vi "LED-Change text.vi"(6 "Container State":T1, 7 "LED Display":refnum<vi>, 8 "error in (no error)":errorcluster, 9 "Should Change?":bool, 10 "Data In":T2, 11 "vi reference in":refnum<vi>) -> (0 "error out":errorcluster, 2 "Data Out":T2, 3 "vi reference out":refnum<vi>)   [LabVIEW 2012, in "LED Display.xctl"]
doc: "This VI changes the text to be displayed in the LED XControl"
uses:
  LED Display.xctl
  LED-Data.ctl
  <vilib>/_xctls/Container State.ctl
  <vilib>/_xctls/XControlSupport.lvlib
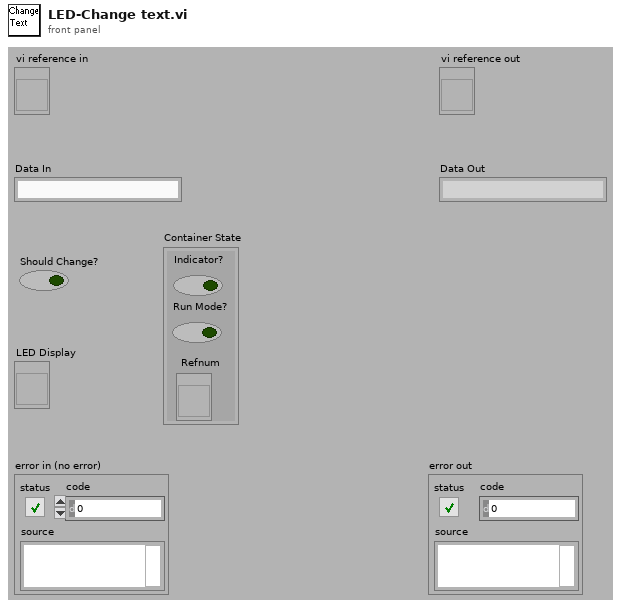
[diagram p1: front panel]
types:
  T1 = typedef "XControlSupport.lvlib/Container State.ctl" = cluster{"Indicator?":bool, "Run Mode?":bool, " Refnum":refnum<vi>}
  T2 = typedef "LED Display.xctl/LED-Data.ctl" = string
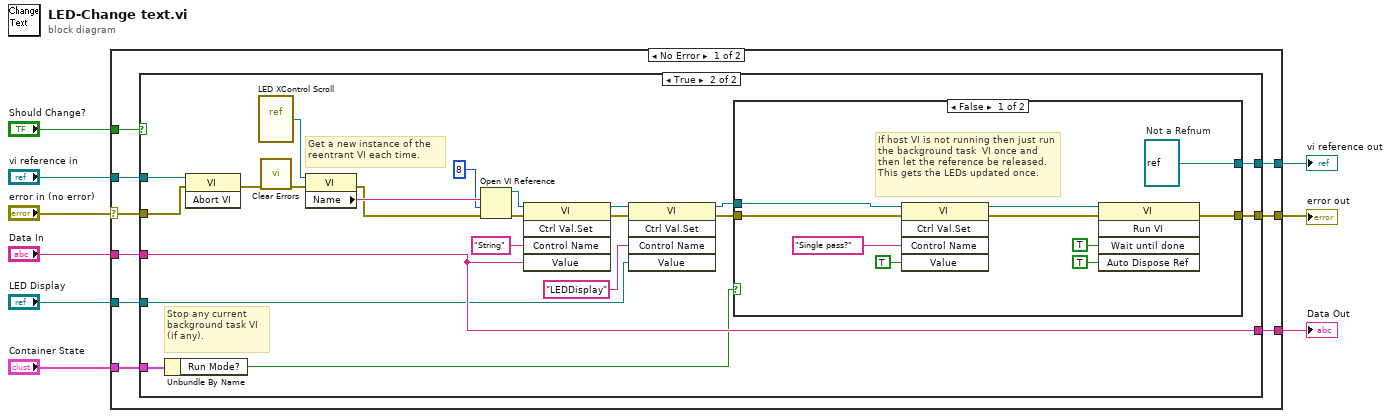
[diagram p0: block diagram]
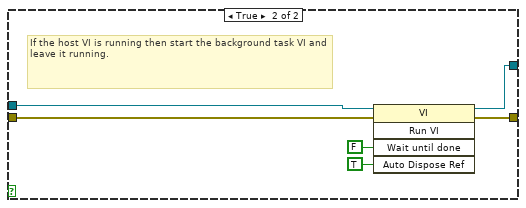
[diagram p3: hidden frame]
diagram:
  n1 = case shown="No Error" "error in (no error)" {
    selector: "error in (no error)" -> [w10 w62]
    tunnel: "LED Display" -> [w18 _]
    tunnel: "Should Change?" -> [w17 _]
    tunnel: "Data In" -> [w16 w60]
    tunnel: [w15 w61] -> w6
    tunnel: [w14 w60] -> w5
    tunnel: "Container State" -> [w13 _]
    tunnel: "vi reference in" -> [w12 w61]
    tunnel: [w11 w62] -> w2
    frame No Error {
      n2 = case shown="True" w17 {
        tunnel: w16 -> [w20 w40]
        tunnel: w12 -> [w21 w43]
        tunnel: [w21 w42] -> w15
        tunnel: w13 -> [_ w41]
        tunnel: [w20 w40] -> w14
        tunnel: w18 -> [_ w39]
        tunnel: [w19 w23] -> w11
        tunnel: w10 -> [w19 w22]
        frame False {
        }
        frame True {
          # "Stop any current\nbackground task VI\n(if any)."
          # "Get a new instance of the \nreentrant VI each time."
          n3 = Unbundle By Name(w41) -> ("Run Mode?"=w38:bool)
          n4 = invoke class="VI" method="Abort VI"(reference=w43, error in=w22) -> (error out=w25:errorcluster)  [unwired: 1 in, 2 out]
          n5 = vi-ref "LED XControl Scroll.vi"() -> (w33:refnum<vi>)
          n6 = call <vilib>:"Clear Errors.vi"("error in (no error)"=w25) -> ("error out"=w26:errorcluster)  [unwired: 6 in]
          n7 = property class="VI"(reference=w33, error in=w26) -> (error out=w24:errorcluster, "Name"=w32:string)  [unwired: 1 out]
          n8 = Open VI Reference(vi path=w32, options=8, error in (no error)=w24) -> (vi reference=w31:refnum<vi>, error out=w27:errorcluster)  [unwired: 3 in]
          n9 = invoke class="VI" method="Ctrl Val.Set"(reference=w31, error in=w27, "Control Name"="String", "Value"=w40) -> (reference out=w36:refnum<vi>, error out=w35:errorcluster)  [unwired: 1 in, 3 out]
          n10 = invoke class="VI" method="Ctrl Val.Set"(reference=w36, error in=w35, "Control Name"="LEDDisplay", "Value"=w39) -> (reference out=w29:refnum<vi>, error out=w28:errorcluster)  [unwired: 1 in, 3 out]
          n11 = case shown="False" w38 {
            tunnel: [w53 w57] -> w42
            tunnel: w29 -> [w49 w56]
            tunnel: w28 -> [w46 w55]
            tunnel: [w44 w54] -> w23
            frame False {
              w53 = refnum<vi> refnum  # Not a Refnum
              # "If host VI is not running then just run the background task  VI once and then let the reference be released. This gets the LEDs updated once."
              n12 = invoke class="VI" method="Ctrl Val.Set"(reference=w49, error in=w46, "Control Name"="Single pass?", "Value"=TRUE ("Auto Dispose Reference")) -> (reference out=w48:refnum<vi>, error out=w47:errorcluster)  [unwired: 1 in, 3 out]
              n13 = invoke class="VI" method="Run VI"(reference=w48, error in=w47, "Wait until done"=TRUE ("Wait Until Done"), "Auto Dispose Ref"=TRUE ("Auto Dispose Reference")) -> (error out=w44:errorcluster)  [unwired: 1 in, 4 out]
            }
            frame True {
              # "If the host VI is running then start the background task VI and leave it running."
              n14 = invoke class="VI" method="Run VI"(reference=w56, error in=w55, "Wait until done"=FALSE ("Wait Until Done"), "Auto Dispose Ref"=TRUE ("Auto Dispose Reference")) -> (reference out=w57:refnum<vi>, error out=w54:errorcluster)  [unwired: 1 in, 3 out]
            }
          }
        }
      }
    }
    frame Error {
    }
  }
  "vi reference out" <- w6
  "Data Out" <- w5
  "error out" <- w2
